vi "Test Cashier Place Order.vi"(8 "error in (no error)":errorcluster, 11 "Cashier Test in":refnum<class "Cashier Test.lvclass">=refnum) -> (0 "error out":errorcluster, 3 "Cashier Test out":refnum<class "Cashier Test.lvclass">)   [LabVIEW 2020, in "Cashier Test.lvclass"]
uses:
  Cashier Test.lvclass
  <vilib>/Astemes/Triarc Framework/Process/Process.lvclass
  Processes/People/Workers/Cashier/Cashier.lvclass
  Processes/People/Workers/Worker/Worker.lvclass
  C:/git/astemes-triarc-examples/source/Coffee Shop/Processes/People/Workers/Worker/Worker.lvclass
  C:/git/astemes-triarc-examples/source/Coffee Shop/Processes/People/Person/Person.lvclass
  C:/Program Files (x86)/National Instruments/LabVIEW 2020/vi.lib/Astemes/Triarc Framework/View/View.lvclass
  C:/Program Files (x86)/National Instruments/LabVIEW 2020/vi.lib/Astemes/Triarc Framework/Process/Process.lvclass
  C:/Program Files (x86)/National Instruments/LabVIEW 2020/vi.lib/Astemes/Triarc Framework/Base/Base.lvclass
  C:/Program Files (x86)/National Instruments/LabVIEW 2020/vi.lib/Astemes/Triarc Framework/Error Handler Interface/Error Handler Interface.lvclass
  C:/Program Files (x86)/National Instruments/LabVIEW 2020/vi.lib/Astemes/Triarc Framework/Logging/Logging.lvclass
  C:/git/astemes-triarc-examples/source/Coffee Shop/Processes/People/Process Job/Job Handler.lvclass
  C:/git/astemes-triarc-examples/source/Coffee Shop/Processes/People/Workers/Cashier/Cashier.lvclass
  <vilib>/Astemes/LUnit/Test Case.lvclass
  Support/Order/Order.lvclass
  Support/Beverages/TypeDefs/Options.ctl
  Support/Beverages/Beverage/Beverage.lvclass
  Support/Beverages/TypeDefs/Drink Type.ctl
  Processes/People/Customers/Customer/Customer.lvclass
  Test Doubles/Mock Job Handler/Mock Job Handler.lvclass
  C:/Program Files (x86)/National Instruments/LabVIEW 2020/vi.lib/Astemes/LUnit/Test Case.lvclass
  C:/Program Files (x86)/National Instruments/LabVIEW 2020/vi.lib/Astemes/LUnit/LUnit Runnable.lvclass
  C:/git/astemes-triarc-examples/source/Coffee Shop/Tests/Test Doubles/Mock Job Handler/Mock Job Handler.lvclass
  Support/Order Item/Order Item.lvclass
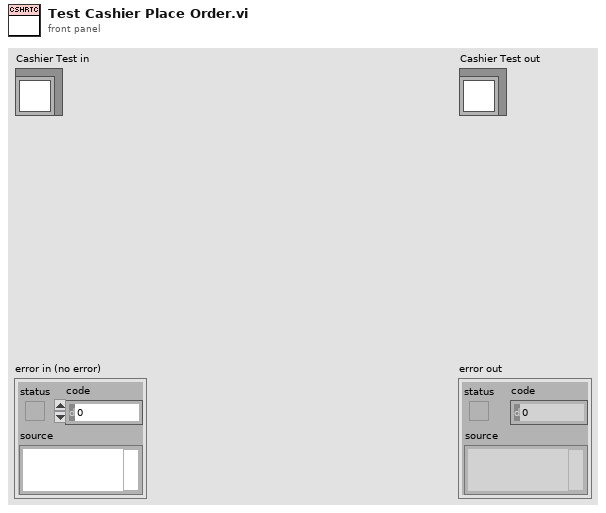
[diagram p1: front panel]
types:
  T1 = typedef "Beverage.lvclass/Drink Type.ctl" = enum16{"Dark Roast", "Decaf", "Espresso", "House Blend"}
  T2 = typedef "Beverage.lvclass/Options.ctl" = enum16{"<None>", "Milk", "Mocha", "Soy", "Whip"}
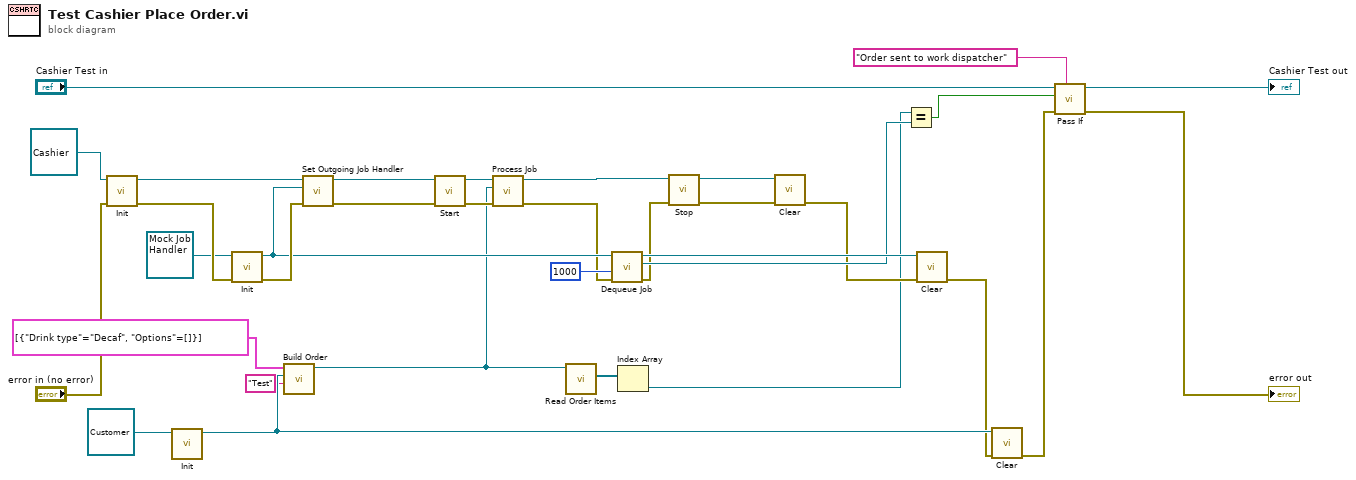
[diagram p0: block diagram]
diagram:
  n1 = call-dynamic "Init.vi"("error in (no error)"="error in (no error)", "View In"=refnum<class "Cashier.lvclass"> refnum ("Cashier.lvclass")) -> ("error out"=w33:errorcluster, "View Out"=w34:refnum<class "Cashier.lvclass">)  [unwired: 8 in]
  n2 = call-dynamic "Init.vi"("View In"=refnum<class "Customer.lvclass"> refnum ("Customer.lvclass")) -> ("View Out"=w11:refnum<class "Customer.lvclass">)  [unwired: 9 in, 1 out]
  n3 = call-dynamic "Init.vi"("error in (no error)"=w33, "Mock Job Handler In"=refnum<class "Mock Job Handler.lvclass"> refnum ("Mock Worker In")) -> ("error out"=w28:errorcluster, "Mock Job Handler Out"=w19:refnum<class "Mock Job Handler.lvclass">)  [unwired: 8 in]
  n4 = call "Build Order.vi"("Customer Name"="Test", "Customer"=w11, "Order"=cluster{"Drink type":T1, "Options":T2[]}[] [{"Drink type"=enum."Decaf", "Options"=[]}]) -> ("Order Out"=w1:refnum<class "Order.lvclass">)  [unwired: 7 in, 1 out]
  n5 = call "Set Outgoing Job Handler.vi"("error in (no error)"=w28, "Work Dispatcher"=w19, "Worker In"=w34) -> ("error out"=w26:errorcluster, "Worker Out"=w27:refnum<class "Cashier.lvclass">)  [unwired: 7 in]
  n6 = call <vilib>:"Start.vi"("error in (no error)"=w26, "Process In"=w27) -> ("error out"=w3:errorcluster, "Process Out"=w5:refnum<class "Cashier.lvclass">)  [unwired: 7 in, 1 out]
  n7 = call-dynamic "Process Job.vi"("error in (no error)"=w3, "Job"=w1, "Worker In"=w5) -> ("error out"=w2:errorcluster, "Worker Out"=w4:refnum<class "Cashier.lvclass">)  [unwired: 7 in]
  n8 = call-dynamic "Read Order Items.vi"("Order in"=w1) -> ("Items"=w8:refnum<class "Order Item.lvclass">[])  [unwired: 8 in, 2 out]
  n9 = call "Dequeue Job.vi"("error in (no error)"=w2, "timeout in ms (-1)"=1000, "Mock Job Handler In"=w19) -> ("error out"=w23:errorcluster, "element"=w25:refnum<class>, "Mock Job Handler Out"=w29:refnum<class "Mock Job Handler.lvclass">)  [unwired: 5 in, 1 out]
  n10 = Index Array(array=w8) -> (element=w7:refnum<class "Order Item.lvclass">)  [unwired: 1 in]
  n11 = call <vilib>:"Stop.vi"("error in (no error)"=w23, "Process In"=w4) -> ("error out"=w31:errorcluster, "Process Out"=w32:refnum<class "Cashier.lvclass">)  [unwired: 7 in, 1 out]
  n12 = call-dynamic "Clear.vi"("error in (no error)"=w31, "View In"=w32) -> ("error out"=w22:errorcluster)  [unwired: 9 in]
  n13 = Equal?(x=w7, y=w25) -> (x = y?=w15:bool)
  n14 = call-dynamic "Clear.vi"("error in (no error)"=w22, "Mock Job Handler In"=w29) -> ("error out"=w10:errorcluster)  [unwired: 9 in]
  n15 = call-dynamic "Clear.vi"("error in (no error)"=w10, "View In"=w11) -> ("error out"=w9:errorcluster)  [unwired: 9 in]
  n16 = call <vilib>:"Pass If.vi"("Description"="Order sent to work dispatcher", "error in (no error)"=w9, "Pass?"=w15, "LUnit Test Case In"="Cashier Test in") -> ("error out"=→"error out":errorcluster, "LUnit Test Case Out"=→"Cashier Test out":refnum<class "Test Case.lvclass">)  [unwired: 6 in]
